vi "ServoControl_myrio_v3_FIFO.vi"() -> ()   [LabVIEW 2019]
uses:
  <vilib>/Platform/TimedLoop/XDataNode/timing_clust.ctl
  <vilib>/Platform/TimedLoop/XDataNode/nitl_modes.ctl
  <vilib>/Platform/TimedLoop/XDataNode/wakeup.ctl
  <vilib>/Instr/_visa.llb/VISA Configure Serial Port (Instr).vi
  <vilib>/Utility/file.llb/Write Delimited Spreadsheet (DBL).vi
  <vilib>/platform/TimedLoop/XDataNode/XDataNode.xnode
  <vilib>/Platform/TimedLoop/XDataNode/XDNodeRunTimeDep.lvlib
panel:
  in  "sinewave amplitude":dbl=8.0 format="%#_13g"
  in  "start FIFO":bool=TRUE
  out "Write FIFO error":errorcluster
  out "# elements write":u32=219
  out "timed out?":bool
  out "rt fifo":refnum<k33>
  in  "Buffer factor":dbl=1.5
  out "# elements read":u32
  out "date/time string":string="1970011"
  out "Create FIFO error":errorcluster
  in  "Experiment Mode":string="20250310_servo_sinewave"
  in  "Times":string="0"
  in  "File Path Control":path=path "C:/Rhex_ABAD"
  in  "const posotion":dbl=180.0
  out "write to visa":string
  out "read from visa":string
  out "sinewave position":dbl
  out "time":dbl
  out "iteration":i32
  in  "const(f)/sine(t)":bool
  in  "graph plot freq.":i32=1
  out "Servo Position Graph":cluster{dbl[], dbl[]}[](graph)
  in  "sinewave period":dbl=10.0
  in  "stop":bool
  in  "Loop Period":i64=5
  in  "VISA resource name":refnum<visa-resource-name>="ASRL2::INSTR"
  in  "baud rate (9600)":u32=500000
  out "error out":errorcluster
  # "Servo motor"
  # "Read data to csv file"
  # "Control botton"
  # "visa setting"
  # "servo setting"
  # "Timed loop status"
  # "FIFO status"
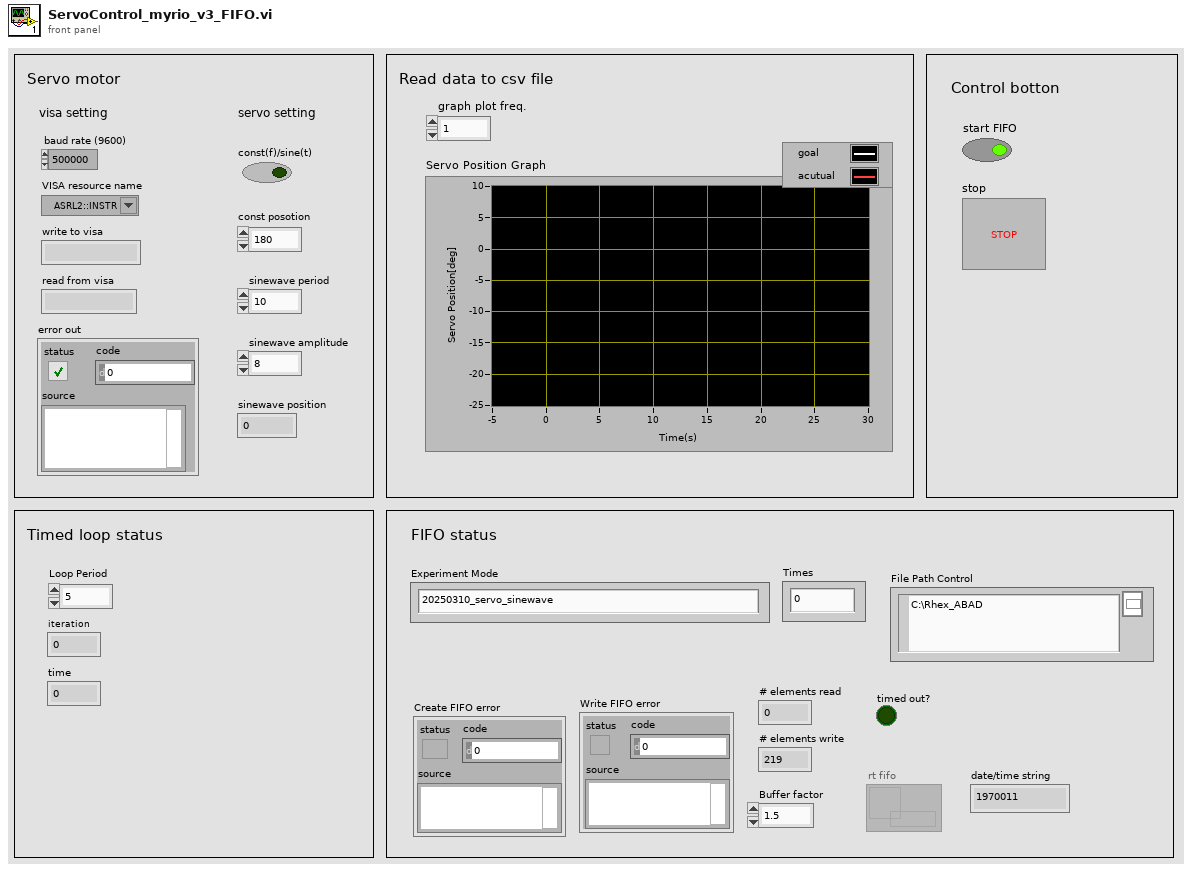
[diagram p1: front panel]
types:
  T1 = typedef "XDNodeRunTimeDep.lvlib/timing_clust.ctl" = cluster{"Expected End [f-1]":u64, "Actual End [f-1]":u64, "Finished Late? [f-1]":bool, "Expected End [i-1]":u64, "Actual End [i-1]":u64, "Finished Late? [i-1]":bool, "Expected Start [i]":u64, "Actual Start [i]":u64, "Expected Start [f]":u64, "Actual Start [f]":u64, "Source Name":string, "Structure Name":string, "Period":i64, "Deadline":i64, "Offset":i64, "Start":i64, "Priority":i32, "Timeout":i32, "Mode":T2, "Wakeup Reason":T3, "Error":errorcluster, "Source Type":string, "Secondary Source Type":string, "Global End Time":u64, "Global Start Time":u64, "Frame Duration":u64, "Iteration Duration":u64, "Assigned CPU":i32, "I/O Scan Engine Mode":u32}
  T2 = typedef "XDNodeRunTimeDep.lvlib/nitl_modes.ctl" = enum32{"No Change", "Process missed periods, maintain original phase", "Discard missed periods, maintain original phase", "Process missed periods, ignore original phase", "Discard missed periods, ignore original phase"}
  T3 = typedef "XDNodeRunTimeDep.lvlib/wakeup.ctl" = enum32{"Normal", "Aborted", "Asynchronous wakeup", "Timing source error", "Timed loop error", "Timeout"}
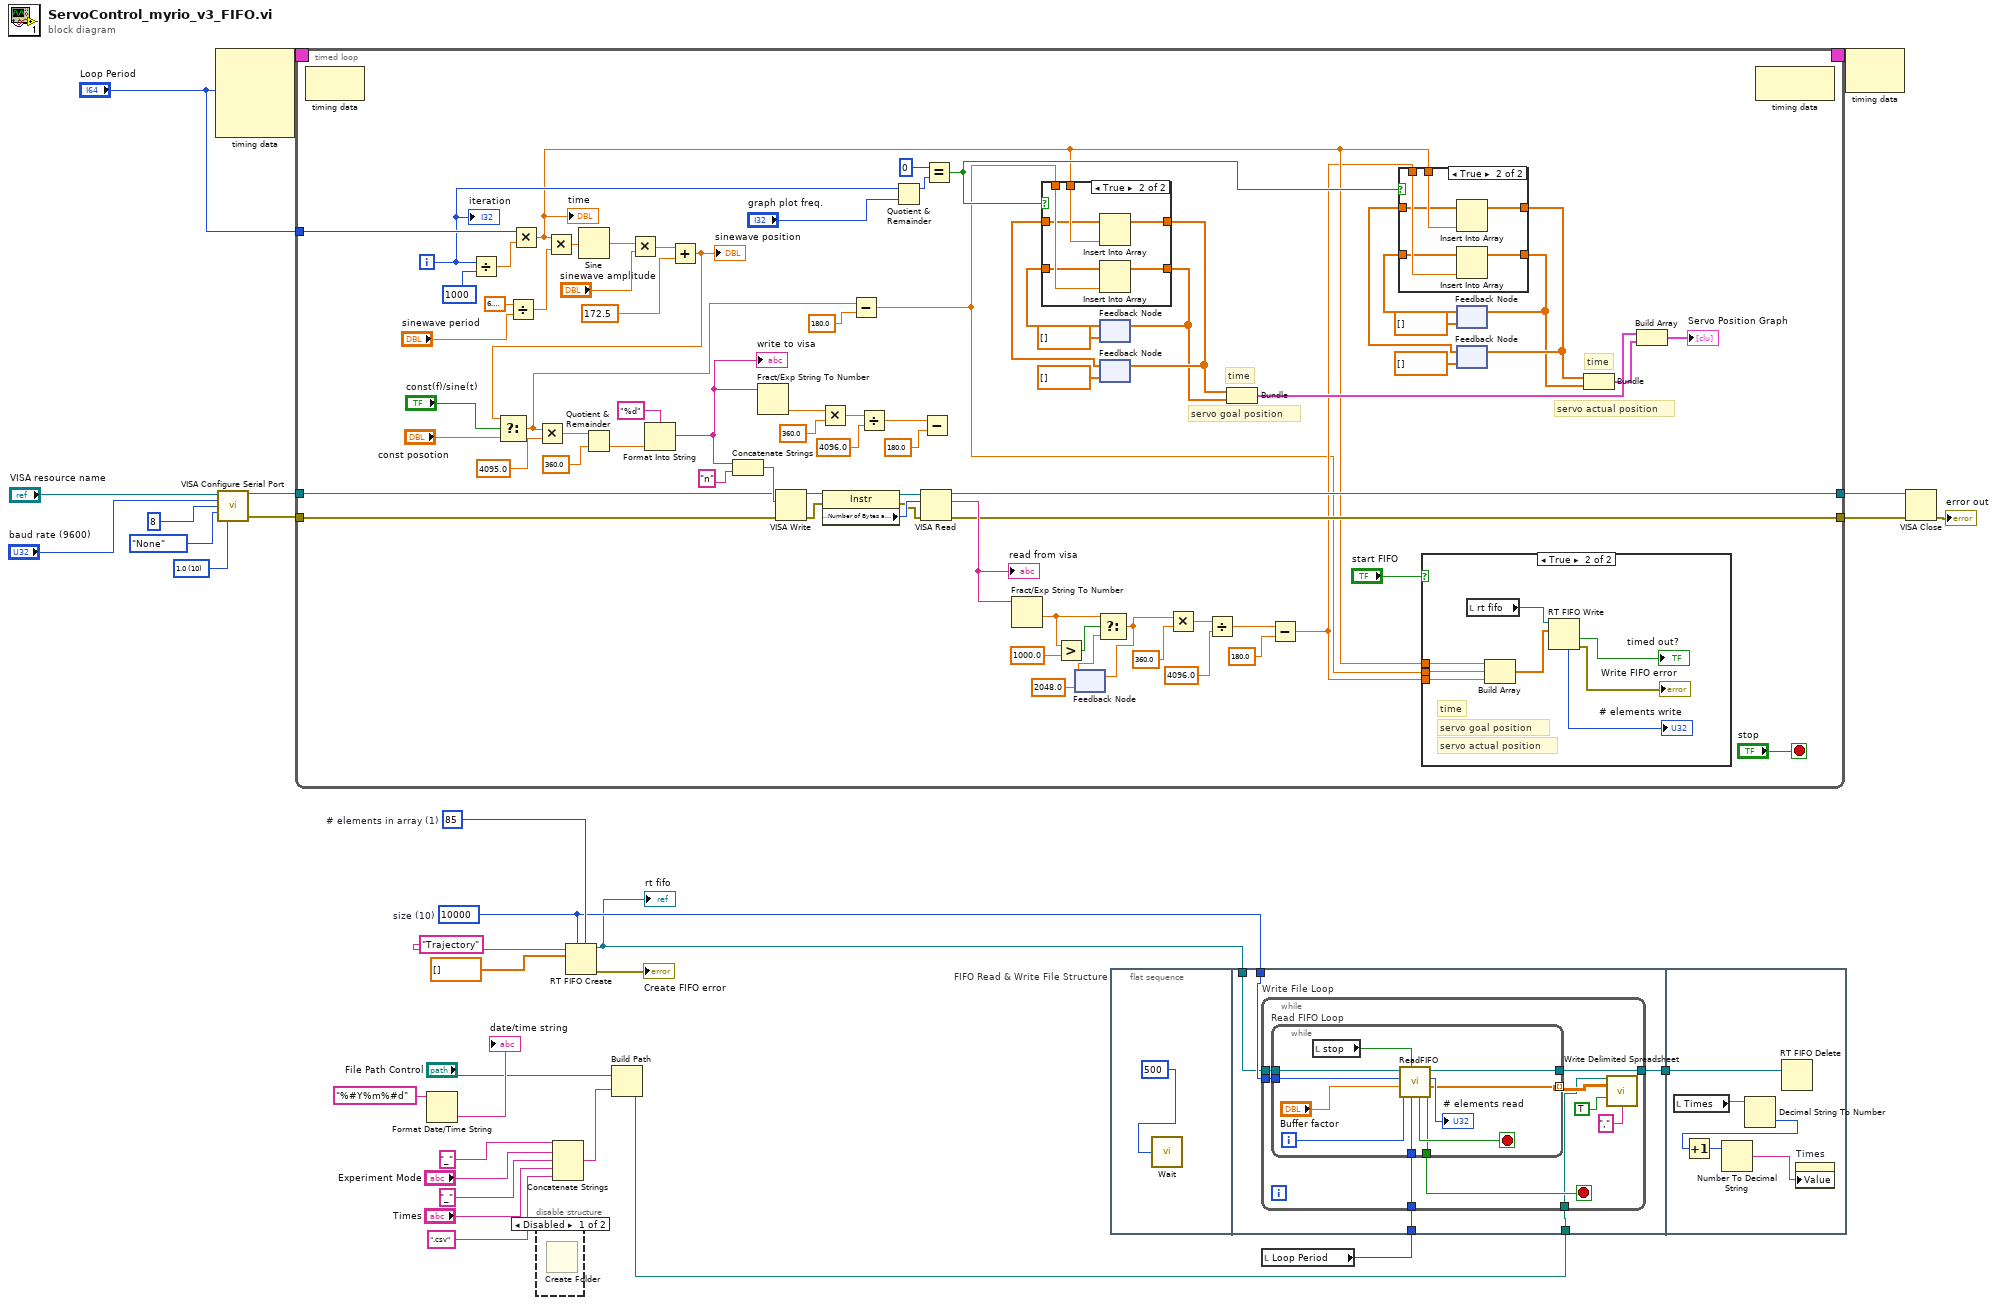
[diagram p0: block diagram]
diagram:
  w7 = u32 85  # # elements in array (1)
  w3 = u32 10000  # size (10)
  w26 = u16 10 items=["1.0"=10, "1.5"=15, "2.0"=20] ("stop bits (10: 1 bit)")
  n1 = node-c288("Loop Period") -> (w31:T1)  [unwired: 3 in]
  n2 = call-poly "VISA Configure Serial Port"("VISA resource name"="VISA resource name", "baud rate (9600)"="baud rate (9600)", "data bits (8)"=u16 8, "parity (0:none)"=enum16{"None", "Odd", "Even", "Mark", "Space"}."None", "stop bits (10: 1 bit)"=w26) -> ("VISA resource name out"=w21:refnum<visa-resource-name>, "error out"=w20:errorcluster)  [unwired: 9 in]
  n3 = timed-loop {
    timing: w31 -> [_]
    timing-out: [_] -> w30
    tunnel: [w46] -> w23
    tunnel: [w45] -> w22
    tunnel: w21 -> [w44]
    tunnel: w20 -> [w43]
    tunnel: "Loop Period" -> [w42]
    i -> [w41]
    stop <- "stop" stop-if-true
    # "time"
    # "servo actual position"
    # "time"
    # "servo goal position"
    n4 = node-c288() -> ()  [unwired: 1 in, 1 out]
    n5 = Divide(x=w41, y=i64 1000) -> (x/y=w86:dbl)
    n6 = Divide(x=6.283185307179586, y="sinewave period") -> (x/y=w50:dbl)
    n7 = Multiply(x=w42, y=w86) -> (x*y=w38:dbl)
    "time" <- w38
    n8 = Multiply(x=w38, y=w50) -> (x*y=w89:dbl)
    n9 = Sine(x=w89) -> (sin(x)=w76:dbl)
    n10 = Multiply(x=w76, y="sinewave amplitude") -> (x*y=w37:dbl)
    n11 = Add(x=w37, y=172.5) -> (x+y=w84:dbl)
    "sinewave position" <- w84
    n12 = Select(t=w84, s="const(f)/sine(t)", f="const posotion") -> (s? t:f=w34:dbl)
    n13 = Multiply(x=w34, y=4095.0) -> (x*y=w105:dbl)
    n14 = Quotient & Remainder(x=w105, y=360.0) -> (floor(x/y)=w103:dbl)  [unwired: 1 out]
    n15 = Format Into String(format string="%d", w103) -> (resulting string=w96:string)  [unwired: 2 in, 1 out]
    "write to visa" <- w96
    n16 = Concatenate Strings(w96, "n" ("string")) -> (w107:string)
    n17 = Fract/Exp String To Number(string=w96) -> (number=w95:dbl)  [unwired: 3 in, 1 out]
    n18 = VISA Write(VISA resource name=w44, write buffer=w107, error in (no error)=w43) -> (VISA resource name out=w74:refnum<visa-resource-name>, error out=w73:errorcluster)  [unwired: 1 out]
    n19 = Multiply(x=w95, y=360.0 ("x")) -> (x*y=w93:dbl)
    n20 = property class="Instr"(reference=w74, error in=w73) -> (reference out=w71:refnum<visa-resource-name>, error out=w70:errorcluster, "Serial Settings:Number of Bytes at Serial Port"=w72:u32)
    n21 = Subtract(x=w34, y=180.0) -> (x-y=w32:dbl)
    n22 = Divide(x=w93, y=4096.0) -> (x/y=w98:dbl)
    n23 = Quotient & Remainder(x=w41, y="graph plot freq.") -> (x-y*floor(x/y)=w79:i32)  [unwired: 1 out]
    n24 = VISA Read(VISA resource name=w71, byte count=w72, error in (no error)=w70) -> (VISA resource name out=w45:refnum<visa-resource-name>, read buffer=w97:string, error out=w46:errorcluster)  [unwired: 1 out]
    "read from visa" <- w97
    n25 = Subtract(x=w98, y=180.0) -> ()  [unwired: 1 out]
    n26 = Equal?(x=0, y=w79) -> (x = y?=w47:bool)
    n27 = Fract/Exp String To Number(string=w97) -> (number=w69:dbl)  [unwired: 3 in, 1 out]
    n28 = Greater?(x=w69, y=1000.0) -> (0:w68:bool)
    n29 = feedback #1(2048.0) -> (w54:dbl)
    n30 = Select(t=w69, s=w68, f=w54) -> (s? t:f=w55:dbl)
    n31 = feedback-in #1(w55) -> ()
    n32 = feedback #2(dbl[] []) -> (w83:dbl[])
    n33 = feedback #3(dbl[] []) -> (w80:dbl[])
    n34 = case shown="True" w47 {
      tunnel: w38 -> [_ w131]
      tunnel: w32 -> [_ w130]
      tunnel: [w125 w129] -> w48
      tunnel: w83 -> [w125 w128]
      tunnel: [w124 w127] -> w49
      tunnel: w80 -> [w124 w126]
      frame False {
      }
      frame True {
        n35 = Insert Into Array(array=w126, new element=w131) -> (w127:dbl[])  [unwired: 1 in]
        n36 = Insert Into Array(array=w128, new element=w130) -> (w129:dbl[])  [unwired: 1 in]
      }
    }
    n37 = feedback-in #2(w48) -> ()
    n38 = feedback-in #3(w49) -> ()
    n39 = Multiply(x=w55, y=360.0 ("x")) -> (x*y=w90:dbl)
    n40 = Divide(x=w90, y=4096.0) -> (x/y=w92:dbl)
    n41 = Bundle(w49, w48) -> (w63:cluster{dbl[], dbl[]})  [unwired: 1 in]
    n42 = Subtract(x=w92, y=180.0) -> (x-y=w36:dbl)
    n43 = case shown="True" "start FIFO" {
      tunnel: w38 -> [_ w110]
      tunnel: w32 -> [_ w109]
      tunnel: w36 -> [_ w108]
      frame False {
      }
      frame True {
        # "time"
        # "servo actual position"
        # "servo goal position"
        n44 = local read "rt fifo"() -> (w112:refnum<k33>)
        n45 = Build Array(w110, w109, w108) -> (w111:dbl[])
        n46 = RT FIFO Write(0:w112, 1:w111) -> (7:→"# elements write":u32, 10:→"timed out?":bool, 11:→"Write FIFO error":errorcluster)  [unwired: 3 in, 1 out]
      }
    }
    n47 = feedback #4(dbl[] []) -> (w67:dbl[])
    n48 = feedback #5(dbl[] []) -> (w64:dbl[])
    n49 = case shown="True" w47 {
      tunnel: w38 -> [_ w123]
      tunnel: w36 -> [_ w122]
      tunnel: [w117 w121] -> w59
      tunnel: w67 -> [w117 w120]
      tunnel: [w116 w119] -> w60
      tunnel: w64 -> [w116 w118]
      frame False {
      }
      frame True {
        n50 = Insert Into Array(array=w118, new element=w123) -> (w119:dbl[])  [unwired: 1 in]
        n51 = Insert Into Array(array=w120, new element=w122) -> (w121:dbl[])  [unwired: 1 in]
      }
    }
    n52 = feedback-in #4(w59) -> ()
    n53 = feedback-in #5(w60) -> ()
    n54 = Bundle(w60, w59) -> (w62:cluster{dbl[], dbl[]})  [unwired: 1 in]
    n55 = Build Array(w63, w62) -> (→"Servo Position Graph":cluster{dbl[], dbl[]}[])
    n56 = node-c288() -> ()  [unwired: 1 in, 1 out]
    "iteration" <- w41
  }
  n57 = Format Date/Time String(time format string (%c)="%#Y%m%#d" ("String 2")) -> (date/time string=→"date/time string":string)  [unwired: 2 in]
  n58 = disable-structure shown="Disabled" {
    frame Disabled {
      n59 = Create Folder() -> ()  [unwired: 3 in, 3 out]
    }
    frame Enabled {
    }
  }
  n60 = Concatenate Strings("_" ("String 2"), "Experiment Mode", "_" ("String 2"), "Times", ".csv" ("string")) -> (w11:string)
  n61 = RT FIFO Create(0:"Trajectory" ("name (unnamed)"), 1:dbl[] [], 4:w3, 6:w7) -> (8:w2:refnum<k33>, 11:→"Create FIFO error":errorcluster)  [unwired: 4 in, 1 out]
  "rt fifo" <- w2
  n62 = Build Path(base path="File Path Control", name or relative path=w11) -> (appended path=w9:path)
  n63 = flat-sequence "FIFO Read & Write File Structure" {
    tunnel: w3 -> [w138]
    tunnel: w1 -> [w137]
    tunnel: w9 -> [w136]
    tunnel: w2 -> [w135]
    tunnel: [w139] -> w18
    tunnel: w18 -> [w160]
    frame #0 {
      n64 = call "Wait"("Count(mSec)"=u32 500 ("Count(uSec)")) -> ()  [unwired: 1 out]
    }
    frame #1 {
      n65 = while "Write File Loop" {
        tunnel: w135 -> [w148]
        tunnel: [w147] -> w139
        tunnel: w138 -> [w146]
        tunnel: w137 -> [w145]
        tunnel: w136 -> [w140]
        stop <- w144 stop-if-true
        n66 = while "Read FIFO Loop" {
          tunnel: w148 -> [w158]
          tunnel: [w152] -> w147
          tunnel: w146 -> [w157]
          tunnel: w145 -> [w155]
          tunnel: [w153] -> w144
          tunnel: [w150] -> w141 mode=indexing
          i -> [w149]
          stop <- w154 stop-if-true
          n67 = local read "stop"() -> (w159:bool)
          n68 = call "ReadFIFO.vi"("dt of Timeloop(ms)"=w155, "Stop"=w159, "Count"=w149, "Buffer factor"="Buffer factor", "FIFO size"=w157, "RT FIFO"=w158) -> ("Stop write file"=w153:bool, "element out"=w150:dbl[], "# elements"=→"# elements read":u32, "RT FIFO (to delete)"=w152:refnum<k33>, "Stop read file"=w154:bool)  [unwired: 1 in]
        }
        n69 = call-poly <vilib>:"Write Delimited Spreadsheet.vi"("file path (dialog if empty)"=w140, "2D data"=w141, "append to file? (new file:F)"=TRUE, "delimiter (\\t)"="," ("delimiter (\\t)")) -> ()  [unwired: 10 in, 2 out]
      }
    }
    frame #2 {
      n70 = local read "Times"() -> (w162:string)
      n71 = Decimal String To Number(string=w162) -> (number=w164:i32)  [unwired: 2 in, 1 out]
      n72 = Increment(x=w164) -> (x+1=w163:i32)
      n73 = Number To Decimal String(number=w163) -> (decimal integer string=w161:string)  [unwired: 1 in]
      n74 = RT FIFO Delete(0:w160) -> ()  [unwired: 2 in, 1 out]
      n75 = property on="Times" class="Str"("Value"=w161) -> ()  [unwired: 2 in, 2 out]
    }
  }
  n76 = local read "Loop Period"() -> (w1:i64)
  n77 = node-c288(w30) -> ()  [unwired: 1 out]
  n78 = VISA Close(VISA resource name=w22, error in (no error)=w23) -> (error out=→"error out":errorcluster)
